vi "EEG_2022_040_LabView_1.3.vi"() -> ()   [LabVIEW 2022 SP3]
panel:
  in  "stop":bool
  in  "Delay Multiplier":dbl(knob) scale=0.0..2.0
  out "Temperature Chart":dbl(graph)
  in  "Number\n of Measurements":dbl
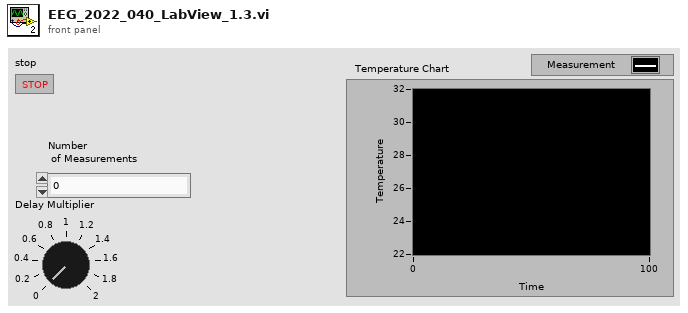
[diagram p1: front panel]
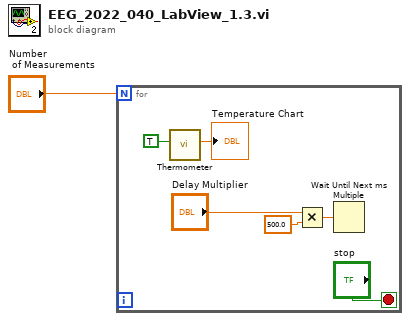
[diagram p0: block diagram]
diagram:
  n1 = for {
    N: "Number\n of Measurements" -> [_]
    stop <- "stop" stop-if-true
    n2 = call "Thermometer.vi"("Temp Scale"=TRUE) -> ("Temperature"=→"Temperature Chart":dbl)  [unwired: 9 in, 1 out]
    n3 = Multiply(x="Delay Multiplier", y=500.0) -> (x*y=w6:dbl)
    n4 = Wait Until Next ms Multiple(millisecond multiple=w6) -> ()  [unwired: 1 out]
  }
